vi "set_array_view_to_last_index_value.vi"(11 "generic array trend_string":string[](array[string])) -> (3 "index":i32[](array[numeric]))   [LabVIEW 2023]
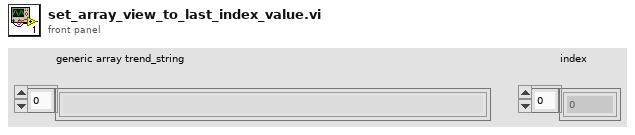
[diagram p1: front panel]
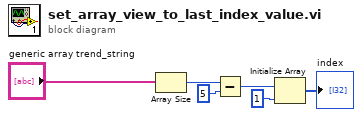
[diagram p0: block diagram]
diagram:
  n1 = Array Size(array="generic array trend_string") -> (size(s)=w5:i32)
  n2 = Subtract(x=w5, y=5) -> (x-y=w4:i32)
  n3 = Initialize Array(w4, 1 ("dimension size")) -> (→"index":i32[])
